vi "Node - PXImc Close.vi"(8 "error in (no error)":errorcluster, 11 "Node Data In":T1) -> (0 "error out":errorcluster, 3 "Node Data Out":T1)   [LabVIEW 2016, in "PXImc Router.lvlib"]
uses:
  PXImc Router.lvlib
  Controls/Node Data.ctl
  <vilib>/NI Veristand/VeriStand Data/Byte Buffer/Byte Buffer.lvclass
  Controls/Node/Node - PXImc Parameters.ctl
  Controls/Node/Transfer Data.ctl
  Controls/Node/Node Ch Properties.ctl
  Controls/Data Type.ctl
  <vilib>/pximc/nipximc.lvlib
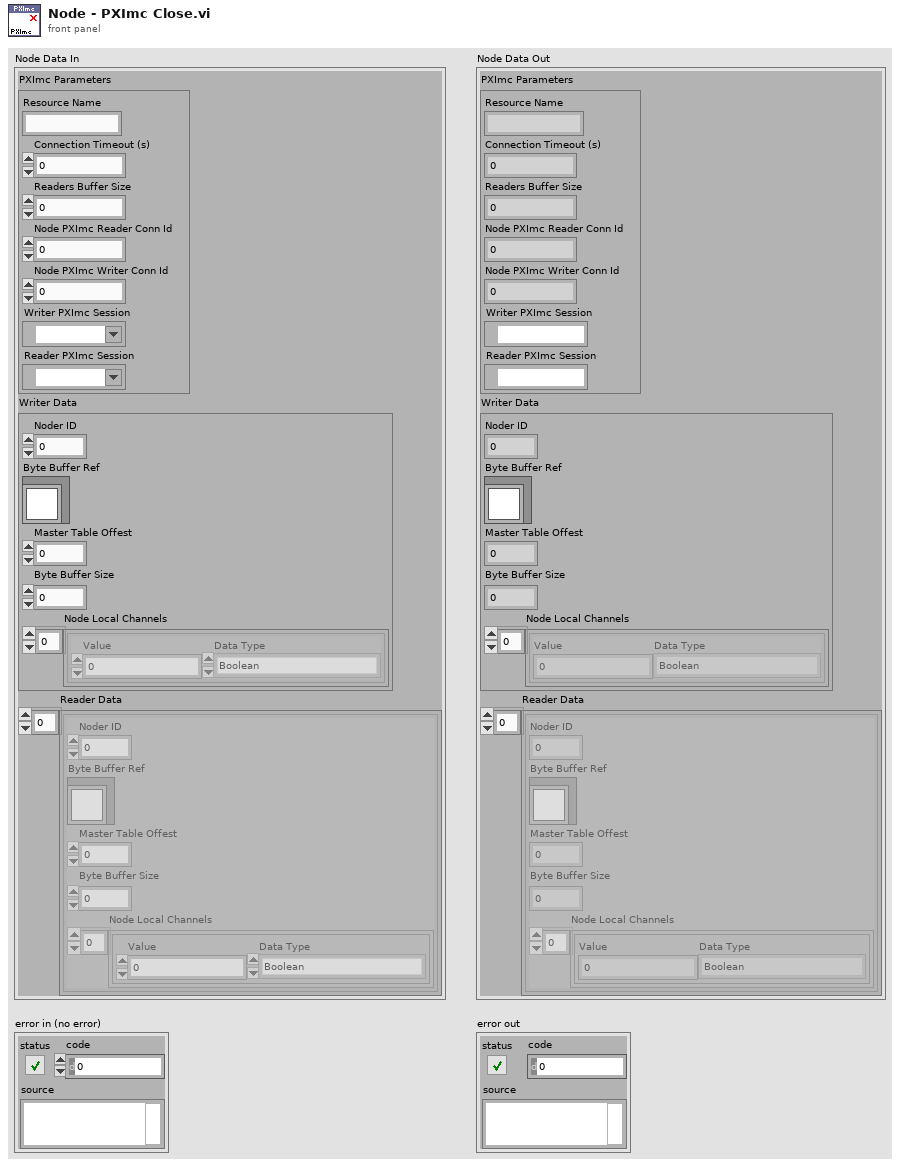
[diagram p1: front panel]
types:
  T1 = typedef "PXImc Router.lvlib/Node Data.ctl" = cluster{"PXImc Parameters":T2, "Writer Data":T3, "Reader Data":T3[]}
  T2 = typedef "PXImc Router.lvlib/Node - PXImc Parameters.ctl" = cluster{"Resource Name":string, "Connection Timeout (s)":dbl, "Readers Buffer Size":u32, "Node PXImc Reader Conn Id":u16, "Node PXImc Writer Conn Id":u16, "Writer PXImc Session":refnum<k21>, "Reader PXImc Session":refnum<k21>}
  T3 = typedef "PXImc Router.lvlib/Transfer Data.ctl" = cluster{"Noder ID":u32, "Byte Buffer Ref":refnum<class "Byte Buffer.lvclass">, "Master Table Offest":u32, "Byte Buffer Size":u32, "Node Local Channels":T4[]}
  T4 = typedef "PXImc Router.lvlib/Node Ch Properties.ctl" = cluster{"Value":dbl, "Data Type":T5}
  T5 = typedef "PXImc Router.lvlib/Data Type.ctl" = enum16{"Boolean", "SGL", "DBL", "I8", "I16", "I32", "I64", "U8", "U16", "U32", "U64"}
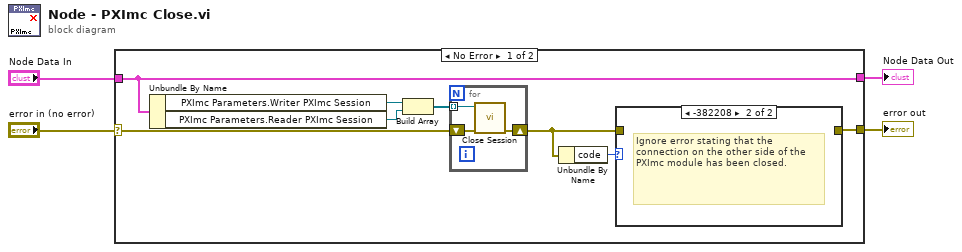
[diagram p0: block diagram]
diagram:
  n1 = case shown="No Error" "error in (no error)" {
    selector: "error in (no error)" -> [w8 w17]
    tunnel: "Node Data In" -> [w12 w18]
    tunnel: [w12 w18] -> w2
    tunnel: [w5 w17] -> w4
    frame No Error {
      n2 = Unbundle By Name(w12) -> ("PXImc Parameters.Writer PXImc Session"=w11:refnum<k21>, "PXImc Parameters.Reader PXImc Session"=w10:refnum<k21>)
      n3 = Build Array(w11, w10) -> (w9:refnum<k21>[])
      n4 = for {
        shift-right: [w15] -> w6
        shift-left: w8 -> [w16]
        tunnel: w9 -> [w14] mode=indexing
        n5 = call <vilib>:"Close Session.vi"("error in (no error)"=w16, "session in"=w14) -> ("error out"=w15:errorcluster)  [unwired: 9 in]
      }
      n6 = Unbundle By Name(w6) -> ("code"=w7:i32)
      n7 = case shown="-382208" w7 {
        tunnel: w6 -> [w13 _]
        tunnel: [w13 _] -> w5
        frame 0, Default {
        }
        frame -382208 {
          # "Ignore error stating that the connection on the other side of the PXImc module has been closed."
        }
      }
    }
    frame Error {
    }
  }
  "error out" <- w4
  "Node Data Out" <- w2
